vi "Notify Observers.vi"(7 "name":string, 8 "error in (no error)":errorcluster, 9 "value":variant, 11 "Observable Actor in":refnum<class "Observable Actor.lvclass">) -> (0 "error out":errorcluster, 3 "Observable Actor out":refnum<class "Observable Actor.lvclass">)   [LabVIEW 2014, in "Observable Actor.lvlib" / "Observable Actor.lvclass"]
uses:
  Observable Actor.lvclass
  Observable Actor.lvclass/Observable Actor.ctl
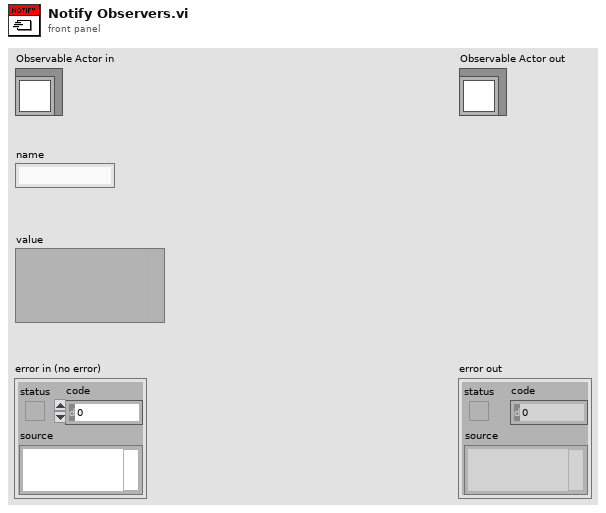
[diagram p1: front panel]
types:
  T1 = typedef "Observable Actor.lvlib/Observable Actor.lvclass/Observer.ctl" = refnum<queue>
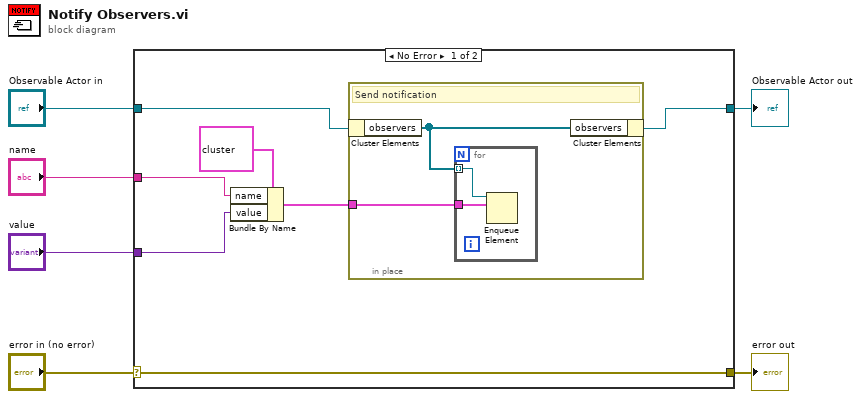
[diagram p0: block diagram]
diagram:
  n1 = case shown="No Error" "error in (no error)" {
    selector: "error in (no error)" -> [w13 w19]
    tunnel: [w13 w19] -> w5
    tunnel: [w8 w18] -> w3
    tunnel: "Observable Actor in" -> [w9 w18]
    tunnel: "name" -> [w11 _]
    tunnel: "value" -> [w10 _]
    frame No Error {
      n2 = Bundle By Name(cluster=cluster{"value":variant, "name":string} {"value"=variant, "name"=""} ("output cluster"), "name"=w11, "value"=w10) -> (w7:cluster{"value":variant, "name":string})
      n3 = in-place {
        in-place-border: w7 -> [w14]
        # "Send notification"
        n4 = in-place-cluster #1(w9) -> ("observers"=w15:T1[])
        n5 = for {
          tunnel: w15 -> [w17] mode=indexing
          tunnel: w14 -> [w16]
          n6 = Enqueue Element(queue=w17, element=w16) -> ()  [unwired: 2 in, 3 out]
        }
        n7 = in-place-cluster #1("observers"=w15) -> (w8:refnum<class "Observable Actor.lvclass">)
      }
    }
    frame Error {
    }
  }
  "error out" <- w5
  "Observable Actor out" <- w3
